vi "Actor Core.vi"(8 "error in":errorcluster, 11 "Panel Form Controller in":refnum<class "Panel Form Controller.lvclass">) -> (0 "error out":errorcluster, 3 "Actor out":refnum<class "Actor.lvclass">)   [LabVIEW 2020, in "Panel Form Controller.lvlib" / "Panel Form Controller.lvclass"]
doc: "The user interface for this panel.\n\n----\nPlease see the following web address for additional documentation and tutorial information:\nhttp://www.mooregoodideas.com/mgi-panel-manager/\n\nAuthor: Derek Trepanier\n\nCopyright (c) 2018, Moore Good Ideas, Inc.\n\nAll rights reserved.\n\nRedistribution and use in source and binary forms, with or without modification, are permitted provided that the following conditions are met:\n\n * Redistributions of source code must retain the above copyright notice, this list of conditions and the following disclaimer.\n * Redistributions in binary form must reproduce the above copyright notice, this list of conditions and the following disclaimer in the documentation and/or other materials provided with the distribution.\n * Neither the name of Moore Good Ideas, Inc. nor the names of its contributors may be used to endorse or promote products derived from this software without specific prior written permission.\n\nTHIS SOFTWARE IS PROVIDED BY THE COPYRIGHT HOLDERS AND CONTRIBUTORS \"AS IS\" AND ANY EXPRESS OR IMPLIED WARRANTIES, INCLUDING, BUT NOT LIMITED TO, THE IMPLIED WARRANTIES OF MERCHANTABILITY AND FITNESS FOR A PARTICULAR PURPOSE ARE DISCLAIMED. IN NO EVENT SHALL THE COPYRIGHT OWNER OR CONTRIBUTORS BE LIABLE FOR ANY DIRECT, INDIRECT, INCIDENTAL, SPECIAL, EXEMPLARY, OR CONSEQUENTIAL DAMAGES (INCLUDING, BUT NOT LIMITED TO, PROCUREMENT OF SUBSTITUTE GOODS OR SERVICES; LOSS OF USE, DATA, OR PROFITS; OR BUSINESS INTERRUPTION) HOWEVER CAUSED AND ON ANY THEORY OF LIABILITY, WHETHER IN CONTRACT, STRICT LIABILITY, OR TORT (INCLUDING NEGLIGENCE OR OTHERWISE) ARISING IN ANY WAY OUT OF THE USE OF THIS SOFTWARE, EVEN IF ADVISED OF THE POSSIBILITY OF SUCH DAMAGE."
uses:
  Panel Form Controller.lvclass
  C:/Program Files (x86)/National Instruments/LabVIEW 2020/vi.lib/MGI/Panel Manager/Panel Actor/Panel Actor/Panel Actor.lvclass
  <vilib>/ActorFramework/Actor/Actor.lvclass
  <vilib>/MGI/Panel Manager/Panel/Panel Helper/Panel Events.ctl
  <vilib>/MGI/Panel Manager/Panel/Panel Helper/Events.ctl
  Panel Form Controller.lvclass/Panel Form Controller.ctl
  <vilib>/ActorFramework/Message Enqueuer/Message Enqueuer.lvclass/Message Enqueuer.ctl
  <vilib>/ActorFramework/Message Enqueuer/Enqueue.vi
  Database OOP/Table Libraries/Basic Form/Basic Form.lvclass
  C:/Users/User/Desktop/Raman Program/Database OOP/source/Database OOP/Table Libraries/Basic Table/Basic Table Class/Basic Table.lvclass
  <vilib>/ActorFramework/Stop Msg/Stop Msg.lvclass
  C:/Program Files (x86)/National Instruments/LabVIEW 2020/vi.lib/ActorFramework/Message/Message.lvclass
  <vilib>/ActorFramework/Message Priority Queue/Priority Enqueue.vi
  <vilib>/MGI/Panel Manager/Panel Actor/Panel Actor/Panel Actor.lvclass
  Database OOP/Table Libraries/Table Configuration Interface/Table Configuration Interface.lvclass
  <vilib>/MGI/Panel Manager/Panel/Panel Helper/Panel Helper.lvclass
  Database OOP/Table Libraries/Basic Table/Basic Table Class/Basic Table.lvclass
types:
  T1 = cluster{"Pnl Actor":refnum<event-registration>, "Child Pnl":refnum<event-registration>, "Child Fields":refnum<event-registration>, "Child Buttons":refnum<event-registration>}
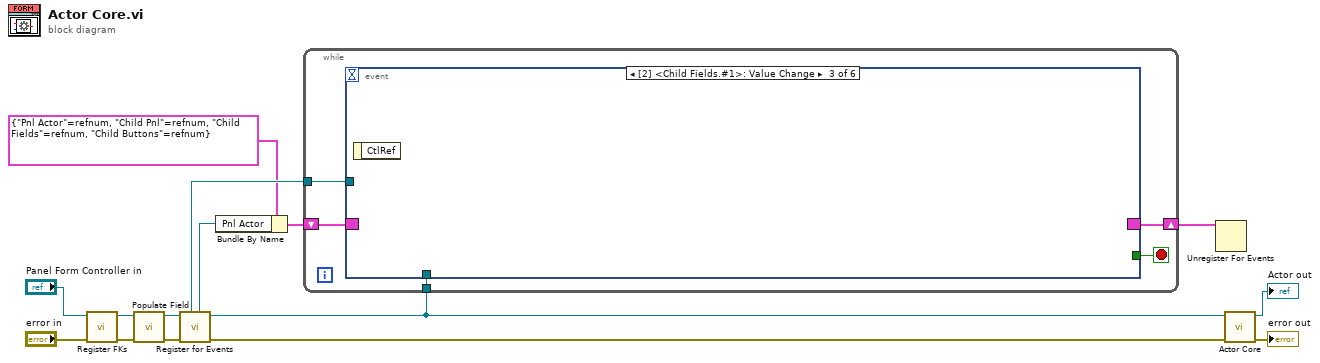
[diagram p0: block diagram]
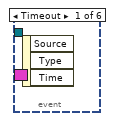
[diagram p2: hidden frame]
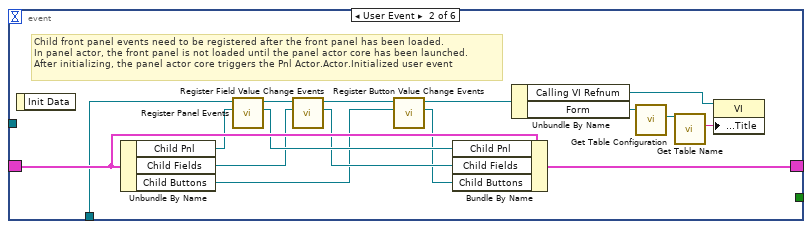
[diagram p3: hidden frame]
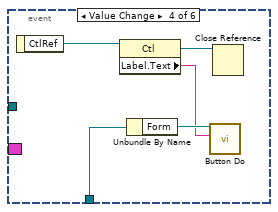
[diagram p4: hidden frame]
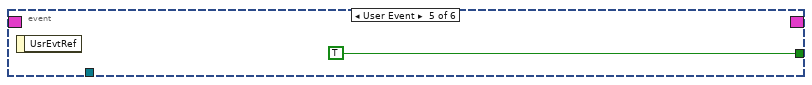
[diagram p5: hidden frame]
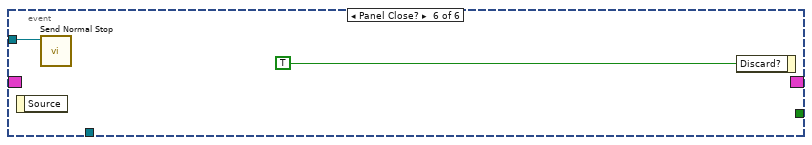
[diagram p6: hidden frame]
diagram:
  n1 = call "Register FKs.vi"("error in (no error)"="error in", "Panel Form Controller in"="Panel Form Controller in") -> ("error out"=w4:errorcluster, "Panel Form Controller out"=w3:refnum<class "Panel Form Controller.lvclass">)  [unwired: 8 in]
  n2 = call "Populate Field.vi"("error in (no error)"=w4, "Panel Form Controller in"=w3) -> ("error out"=w5:errorcluster, "Panel Form Controller out"=w6:refnum<class "Panel Form Controller.lvclass">)  [unwired: 8 in]
  n3 = call <vilib>:"Register for Events.vi"("Error In"=w5, "Panel Actor in"=w6) -> ("Error Out"=w8:errorcluster, "Panel Actor out"=w7:refnum<class "Panel Form Controller.lvclass">, "Pnl Actor"=w9:refnum<event-registration>, "Self Enqueuer"=w12:refnum<class "Message Enqueuer.lvclass">)  [unwired: 6 in]
  n4 = Bundle By Name(cluster=T1 {"Pnl Actor"=refnum, "Child Pnl"=refnum, "Child Fields"=refnum, "Child Buttons"=refnum}, "Pnl Actor"=w9) -> (w10:T1)
  n5 = while {
    tunnel: w12 -> [w20]
    tunnel: w7 -> [w16]
    shift-right: [w18] -> w13
    shift-left: w10 -> [w17]
    stop <- w19 stop-if-true
    n6 = event shown="[2] <Child Fields.#1>: Value Change" {
      selector: w17 -> [_ w36 _ _ _ _]
      dyn-events: [_ w35 _ _ _ _] -> w18
      timeout: _ -> [_ _ _ _ _ _]
      tunnel: w20 -> [_ _ _ _ _ w44]
      tunnel: [_ _ _ _ TRUE _] -> w19
      tunnel: w16 -> [_ w29 _ w40 _ _]
      event Timeout {
        n7 = event-data() -> ()  [unwired: 1 in, 3 out]
      }
      event User Event {
        # "Child front panel events need to be registered after the front panel has been loaded.\nIn panel actor, the front panel is not loaded until the panel actor core has been launched.\nAfter initializing, the panel actor core triggers the Pnl Actor.Actor.Initialized user event"
        n8 = event-data() -> ()  [unwired: 1 in, 1 out]
        n9 = Unbundle By Name(w36) -> ("Child Pnl"=w34:refnum<event-registration>, "Child Fields"=w32:refnum<event-registration>, "Child Buttons"=w27:refnum<event-registration>)
        n10 = call "Register Panel Events.vi"("Event Refnum In"=w34, "Panel Form Controller in"=w29) -> ("Event Refnum Out"=w33:refnum<event-registration>, "Panel Form Controller out"=w30:refnum<class "Panel Form Controller.lvclass">)  [unwired: 7 in, 1 out]
        n11 = call "Register Field Value Change Events.vi"("Field Event Refnum In"=w32, "Panel Form Controller in"=w30) -> ("Field Event Refnum Out"=w31:refnum<event-registration>, "Panel Form Controller out"=w28:refnum<class "Panel Form Controller.lvclass">)  [unwired: 7 in, 1 out]
        n12 = call "Register Button Value Change Events.vi"("Button Event Refnum In"=w27, "Panel Form Controller in"=w28) -> ("Button Event Refnum Out"=w26:refnum<event-registration>, "Panel Form Controller out"=w25:refnum<class "Panel Form Controller.lvclass">)  [unwired: 7 in, 1 out]
        n13 = Bundle By Name(cluster=w36, "Child Pnl"=w33, "Child Fields"=w31, "Child Buttons"=w26) -> (w35:T1)
        n14 = Unbundle By Name(w25) -> ("Calling VI Refnum"=w21:refnum<vi>, "Form"=w24:refnum<class "Basic Form.lvclass">)
        n15 = call "Get Table Configuration.vi"("Basic Table in"=w24) -> ("Table Configuration"=w23:refnum<class "Table Configuration Interface.lvclass">)  [unwired: 8 in, 2 out]
        n16 = call-dynamic "Get Table Name.vi"("Table Configuration Interface in"=w23) -> ("Table Name"=w22:string)  [unwired: 8 in, 2 out]
        n17 = property class="VI"(reference=w21, "Front Panel.Title"=w22) -> ()  [unwired: 1 in, 2 out]
      }
      event Value Change {
        n18 = event-data() -> ()  [unwired: 1 in, 1 out]
      }
      event Value Change {
        n19 = event-data() -> ("CtlRef"=w41:refnum<vi>)  [unwired: 1 in]
        n20 = property class="Ctl"(reference=w41) -> (reference out=w37:refnum<vi>, "Label.Text"=w38:string)  [unwired: 1 in, 1 out]
        n21 = Unbundle By Name(w40) -> ("Form"=w39:refnum<class "Basic Form.lvclass">)
        n22 = call "Button Do.vi"("Button Name"=w38, "Basic Form in"=w39) -> ()  [unwired: 8 in, 2 out]
        n23 = Close Reference(reference=w37) -> ()  [unwired: 1 in, 1 out]
      }
      event User Event {
        n24 = event-data() -> ()  [unwired: 1 in, 1 out]
      }
      event Panel Close? {
        n25 = event-data() -> ()  [unwired: 1 in, 1 out]
        n26 = call <vilib>:"Send Normal Stop.vi"("Message Enqueuer"=w44) -> ()  [unwired: 10 in, 1 out]
        n27 = event-data("Discard?"=TRUE) -> ()  [unwired: 1 in, 1 out]
      }
    }
  }
  n28 = Unregister For Events(event registration refnum=w13) -> ()  [unwired: 1 in, 1 out]
  n29 = call-parent "Actor Core.vi"("error in"=w8, "Panel Actor in"=w7) -> ("error out"=→"error out":errorcluster, "Actor out"=→"Actor out":refnum<class "Actor.lvclass">)  [unwired: 8 in]
